vi "TestServo.vi"   [LabVIEW 2012]
types:
  T1 = typedef "URAPI_Control.ctl" = cluster{"Script":string, "Whiles":u8[], "Ifs":u8[], "Supress Err":bool, "Errors":string}
  T2 = typedef "URAPI_Control.ctl" = cluster{"Script":string, "Whiles":u8[], "Ifs":u8[], "remote":bool, "RIO Settings":T3, "Supress Err":bool}
  T3 = typedef "RIO_Control.ctl" = cluster{"IP Address":string, "Connected?":bool, "connection ID":refnum<k5>, "Script":string}
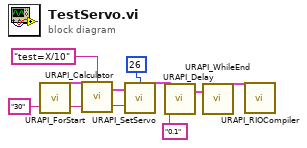
[diagram p0: block diagram]
diagram:
  n1 = call <userlib>:"URAPI_ForStart.vi"("Iterations"="30") -> ("variable"=w11:string, "URAPI Script Out"=w10:T1)  [unwired: 3 in]
  n2 = call <userlib>:"URAPI_Calculator.vi"("X"=w11, "URAPI Script"=w10, "Formula"="test=X/10") -> ("Variable Out"=w9:string, "URAPI Script"=w8:T2)  [unwired: 1 in]
  n3 = call <userlib>:"URAPI_SetServo.vi"("Variable In"=w9, "URAPI Script"=w8, "Port"=26) -> ("URAPI Script"=w3:T2)  [unwired: 1 in, 1 out]
  n4 = call <userlib>:"URAPI_Delay.vi"("Variable In"="0.1", "URAPI Script"=w3) -> ("URAPI Script out"=w2:T1)  [unwired: 3 in]
  n5 = call <userlib>:"URAPI_WhileEnd.vi"("URAPI Script"=w2) -> ("URAPI Script Out"=w5:T1)  [unwired: 4 in]
  n6 = call <userlib>:"URAPI_RIOCompiler.vi"("URAPI Script"=w5) -> ()  [unwired: 4 in, 1 out]
